vi "Vision Processing.vi"(4 "error in (no error)":errorcluster) -> ()   [LabVIEW 2012]
doc: "This VI runs in parallel to other tasks. It gets images from the camera, processes them for color or shape and use that information to affect robot behavior."
uses:
  Robot Global Data.vi
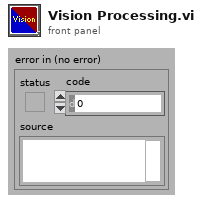
[diagram p1: front panel]
types:
  T1 = typedef "Image Type" = u32
  T2 = typedef "WPI_CameraDevRef.ctl" = cluster{"Camera Address":string, "CameraStatus":errorcluster, "Acquire Image Notifier":refnum<notifier>}
  T3 = typedef "IMAQ Image.ctl" = refnum<image>
  T4 = typedef "WPI_CameraImageSize.ctl" = enum16{"640x480", "320x240", "160x120"}
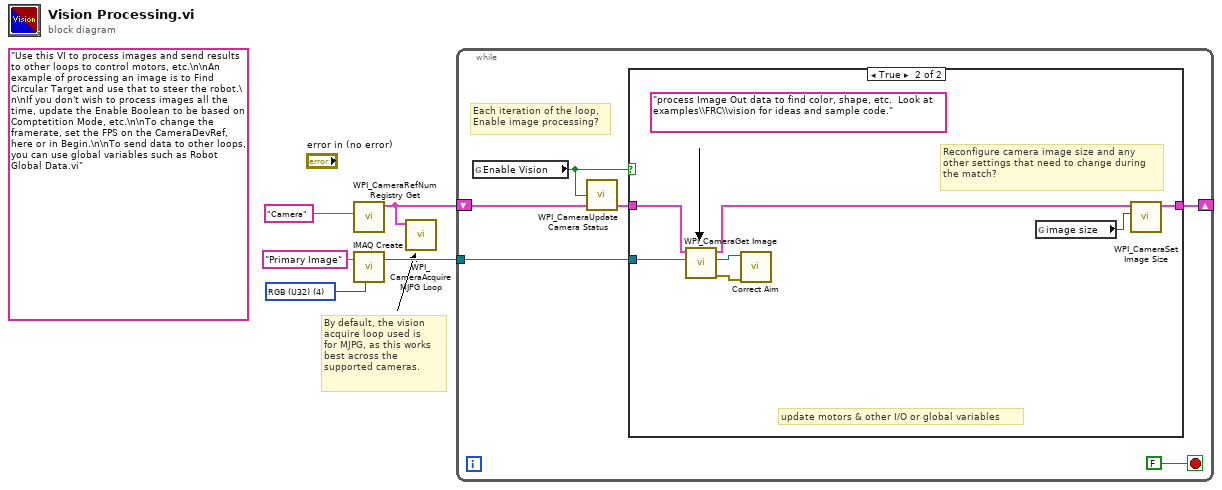
[diagram p0: block diagram]
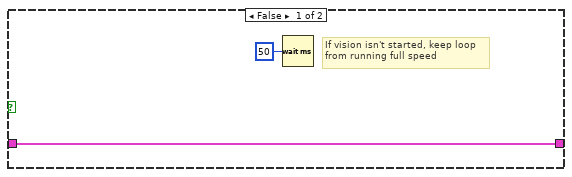
[diagram p2: hidden frame]
diagram:
  (unwired) "Use this VI to process images and send results to other loops to control motors, etc.\n\nAn example of processing an image is to Find Circular Target and use that to steer the robot.\n\nIf you don't wish to process images all the time, update the Enable Boolean to be based on Comptetition Mode, etc.\n\nTo change the framerate, set the FPS on the CameraDevRef, here or in Begin.\n\nTo send data to other loops, you can use global variables such as Robot Global Data.vi"
  w5 = T1 4 items=["Grayscale (U8)", "Grayscale (I16)", "Grayscale (SGL)", "Complex (CSG)", "RGB (U32)", "HSL (U32)", "RGB (U64)"] ("Image Type")
  # "By default, the vision\nacquire loop used is\nfor MJPG, as this works\nbest across the\nsupported cameras."
  n1 = call <vilib>:"WPI_CameraRefNum Registry Get.vi"("refnum name"="Camera") -> ("CameraDevRef"=w1:T2)  [unwired: 1 in, 9 out]
  n2 = call "IMAQ Create"("Image Name"="Primary Image", "Image Type"=w5) -> ("New Image"=w3:T3)  [unwired: 2 in, 2 out]
  n3 = call <vilib>:"WPI_CameraAcquire MJPG Loop.vi"("CameraDevRef"=w1) -> ()  [unwired: 11 in]
  n4 = while {
    shift-right: [w10] -> _
    shift-left: w1 -> [w8]
    tunnel: w3 -> [w9]
    stop <- FALSE stop-if-true
    # "Each iteration of the loop,\nEnable image processing?"
    n5 = global read "Robot Global Data.vi" "Enable Vision"() -> (w6:bool)
    n6 = call <vilib>:"WPI_CameraUpdate Camera Status.vi"("CameraDevRef In"=w8, "Enable Vision"=w6) -> ("CameraDevRef Out"=w7:T2)  [unwired: 3 in]
    n7 = case shown="True" w6 {
      tunnel: w9 -> [_ w19]
      tunnel: [w13 w20] -> w10
      tunnel: w7 -> [w13 w17]
      frame False {
        # "If vision isn't started, keep loop\nfrom running full speed"
        n8 = Wait (ms)(milliseconds to wait=u32 50) -> ()  [unwired: 1 out]
      }
      frame True {
        (unwired) "process Image Out data to find color, shape, etc.  Look at examples\\FRC\\vision for ideas and sample code."
        # "update motors & other I/O or global variables"
        # "Reconfigure camera image size and any\nother settings that need to change during\nthe match?"
        n9 = call <vilib>:"WPI_CameraGet Image.vi"("Image"=w19, "CameraDevRef"=w17) -> ("error out"=w15:errorcluster, "Image Out"=w14:T3, "CameraDevRef Out"=w16:T2)  [unwired: 1 in, 6 out]
        n10 = call "Correct Aim.vi"("error in"=w15, "Image In"=w14) -> ()  [unwired: 8 in, 2 out]
        n11 = global read "Robot Global Data.vi" "image size"() -> (w18:T4)
        n12 = call <vilib>:"WPI_CameraSet Image Size.vi"("Image Size"=w18, "CameraDevRef"=w16) -> ("CameraDevRef Out"=w20:T2)  [unwired: 1 in, 8 out]
      }
    }
  }
